vi "状态机的使用(上).vi"() -> ()   [LabVIEW 2018]
panel:
  out "当前时刻状态":enum16{"111", "110", "101", "001", "000"}(ring)
  in  "布尔":bool
  in  "枚举":enum16{"111", "110", "101", "001", "000"}(ring)
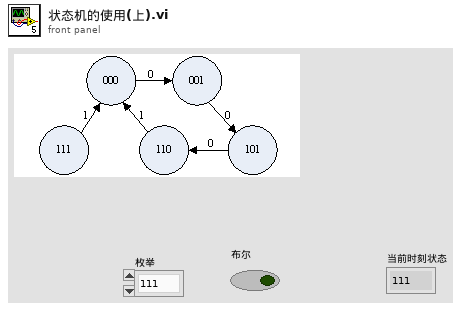
[diagram p1: front panel]
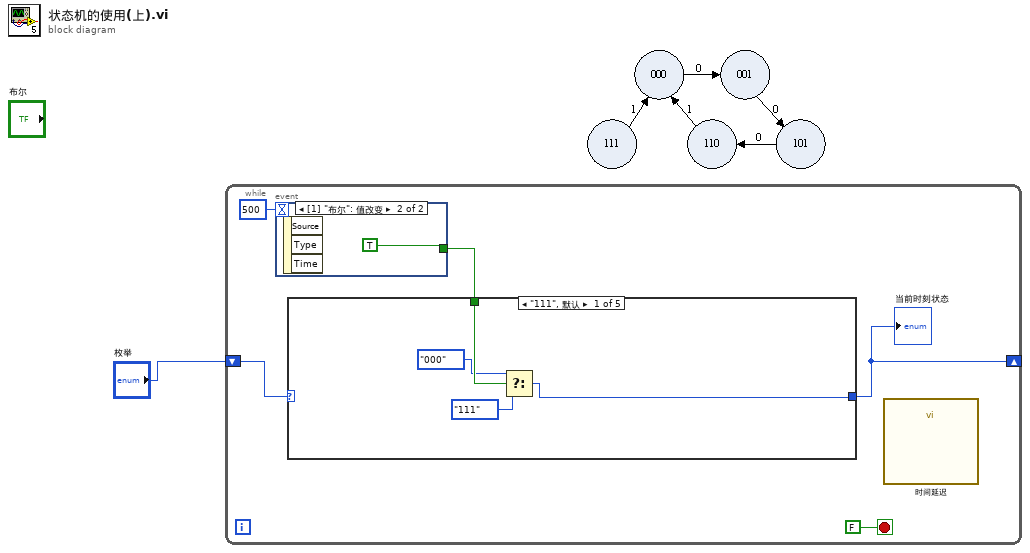
[diagram p0: block diagram]
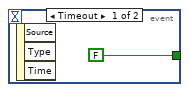
[diagram p2: hidden frame]
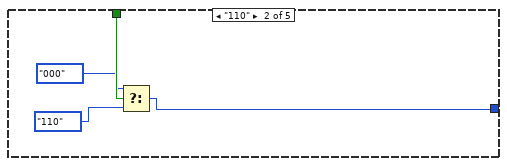
[diagram p3: hidden frame]
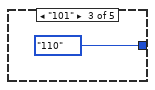
[diagram p4: hidden frame]
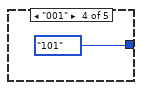
[diagram p5: hidden frame]
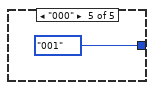
[diagram p6: hidden frame]
diagram:
  n1 = while {
    shift-right: [w4] -> _
    shift-left: "枚举" -> [w5]
    stop <- FALSE stop-if-true
    n2 = event shown="[1] \"布尔\": 值改变" {
      selector: _ -> [_ _]
      dyn-events: _ -> [_ _]
      timeout: 500 -> [_ _]
      tunnel: [FALSE TRUE] -> w2
      event Timeout {
        n3 = event-data() -> ()  [unwired: 1 in, 3 out]
      }
      event "布尔": Value Change {
        n4 = event-data() -> ()  [unwired: 1 in, 3 out]
      }
    }
    n5 = case shown="\"111\", 默认" w5 {
      tunnel: [w9 w13 enum16{"111", "110", "101", "001", "000"}."110" ("枚举") enum16{"111", "110", "101", "001", "000"}."101" ("枚举") enum16{"111", "110", "101", "001", "000"}."001" ("枚举")] -> w4
      tunnel: w2 -> [w12 w16 _ _ _]
      frame "111", Default {
        n6 = Select(t=enum16{"111", "110", "101", "001", "000"}."000" ("枚举"), s=w12, f=enum16{"111", "110", "101", "001", "000"}."111" ("枚举")) -> (s? t:f=w9:enum16{"111", "110", "101", "001", "000"})
      }
      frame "110" {
        n7 = Select(t=enum16{"111", "110", "101", "001", "000"}."000" ("枚举"), s=w16, f=enum16{"111", "110", "101", "001", "000"}."110" ("枚举")) -> (s? t:f=w13:enum16{"111", "110", "101", "001", "000"})
      }
      frame "101" {
      }
      frame "001" {
      }
      frame "000" {
      }
    }
    "当前时刻状态" <- w4
    n8 = call "时间延迟"() -> ()  [unwired: 11 in, 1 out]
  }
